vi "Main.vi"(8 "error in":errorcluster, 11 "Test Timer in":refnum<class "Test Timer.lvclass">) -> (0 "error out":errorcluster, 3 "Test Timer out":refnum<class "Test Timer.lvclass">)   [LabVIEW 2021, in "Test Timer.lvclass"]
doc: "The <b>Queued Message Handler</b> of the Worker that owns this VI."
uses:
  Test Timer.lvclass
  Test Timer.lvclass/Test Timer.ctl
  Initialization Data.ctl
  Response Cases.ctl
  Utility/Utility.lvlib
  Timer/Timer.lvclass
  <vilib>/addons/_Workers/Library/Case Label.ctl
  <vilib>/addons/_Workers/Library/Workers.lvlib
  Timer/rqp_Start.ctl
panel:
  in  "Exit":bool
  in  "Abort Timer":bool
  out "Response 2 recieved":i32
  out "Response 1 recieved":i32
  in  "Response case Test Timer":enum16{"Response 1", "Response 2"}(ring)
  in  "# Copies (0 = infinite repeat)":i32=3
  in  "Period [ms]":i32=1000 min=20
  in  "Start":bool
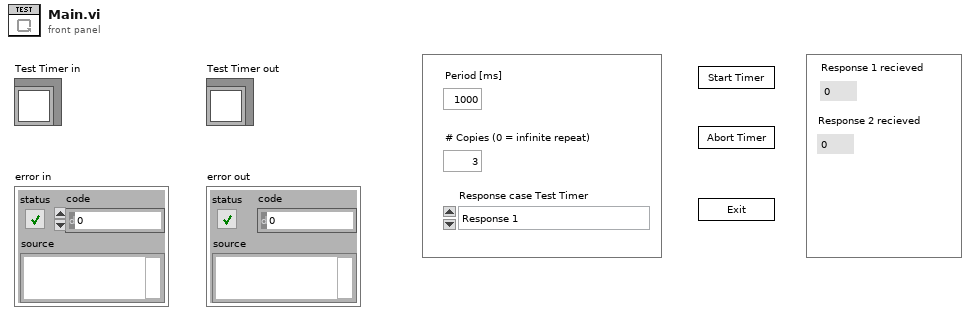
[diagram p1: front panel]
types:
  T1 = enum32{"Invalid", "Standard", "Closed", "Hidden", "Minimized", "Maximized"}
  T2 = typedef "Test Timer.lvclass/Initialization Data.ctl" = cluster{"Response Cases":T3}
  T3 = typedef "Test Timer.lvclass/Response Cases.ctl" = cluster{"Placeholder - Can be deleted":string}
  T4 = typedef "Timer.lvclass/rqp_Start.ctl" = cluster{"Timeout (ms)":i32, "# Copies":i32, "Response Case":T5}
  T5 = typedef "Workers.lvlib/Case Label.ctl" = string
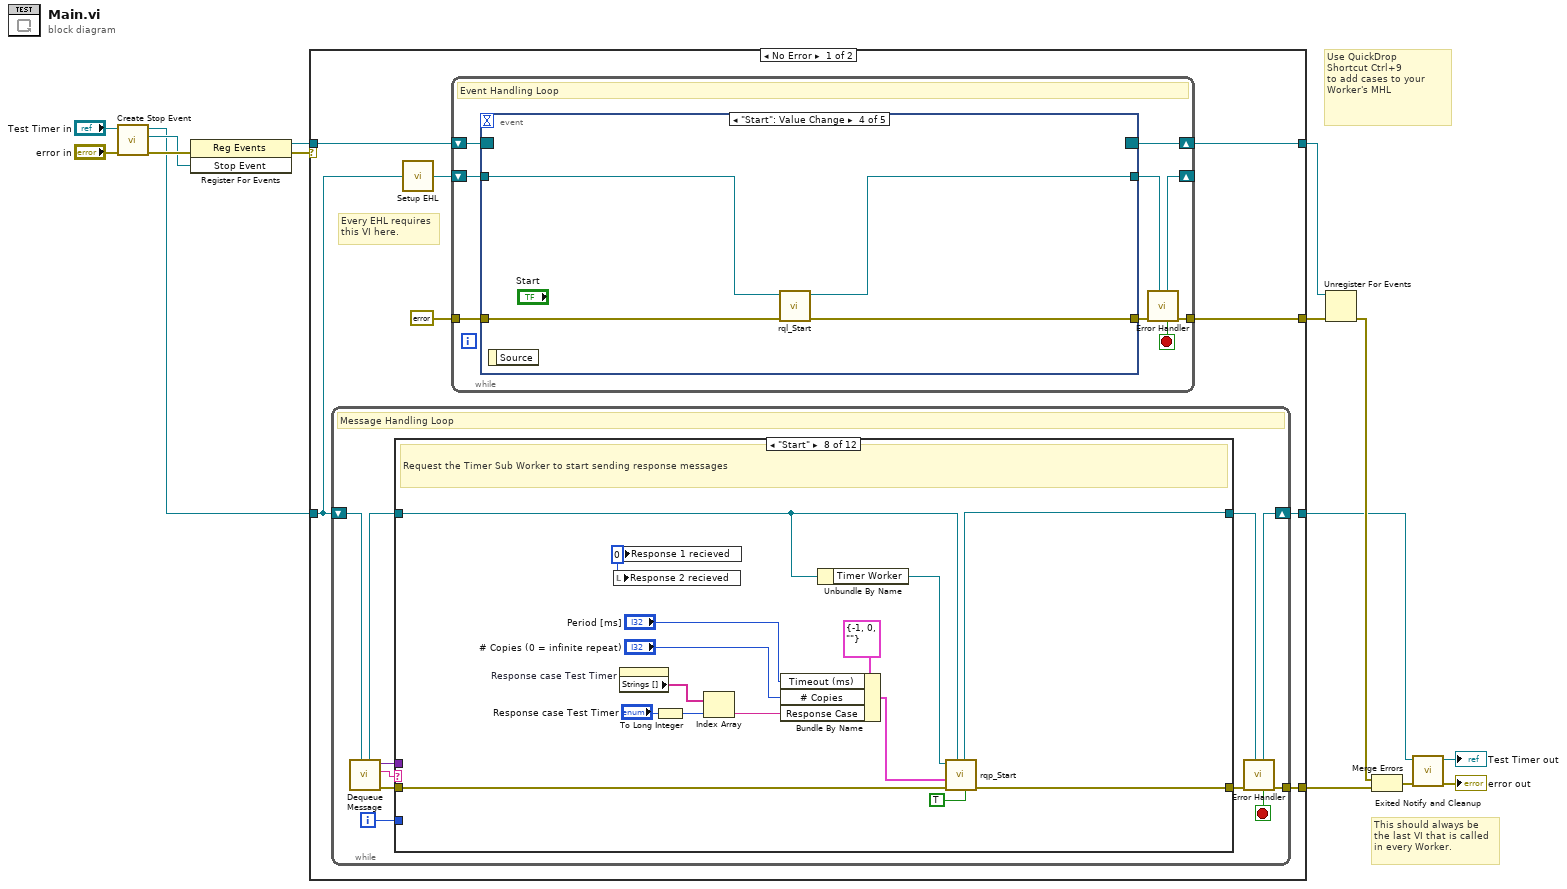
[diagram p0: block diagram]
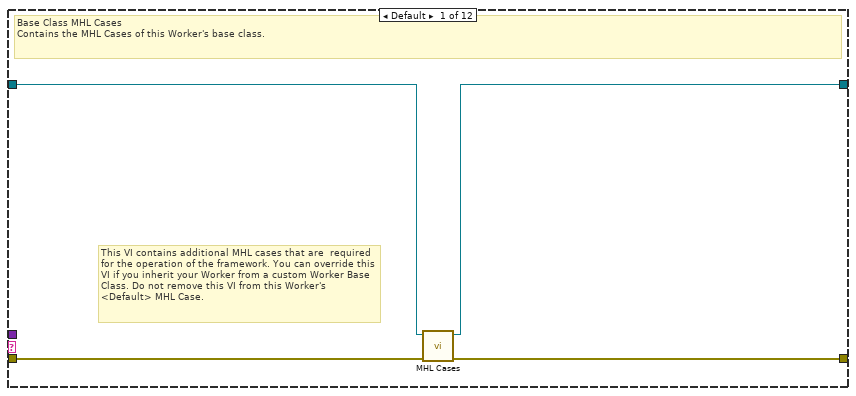
[diagram p2: hidden frame]
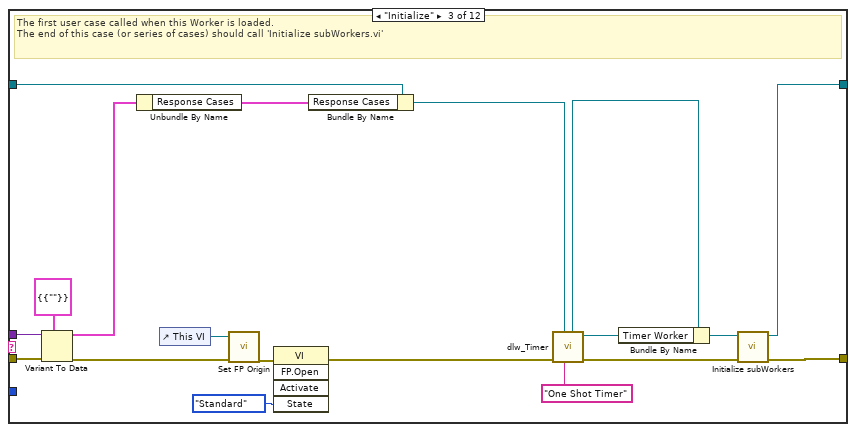
[diagram p4: hidden frame]
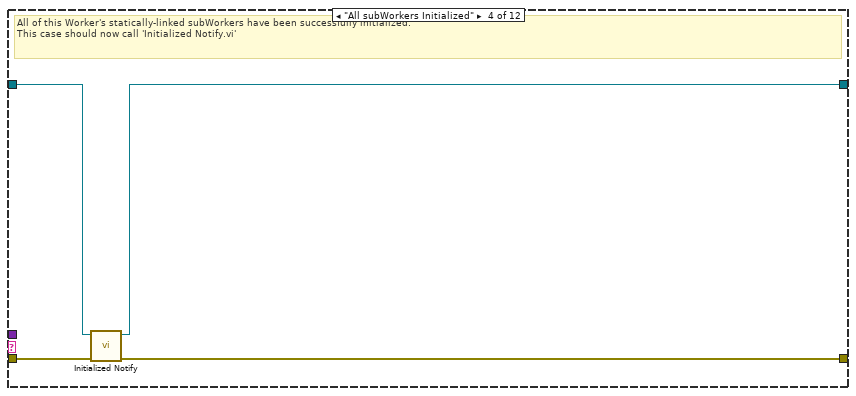
[diagram p5: hidden frame]
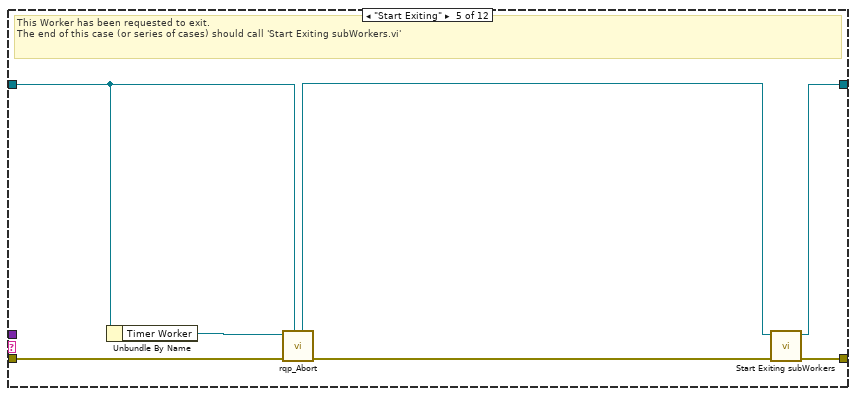
[diagram p6: hidden frame]
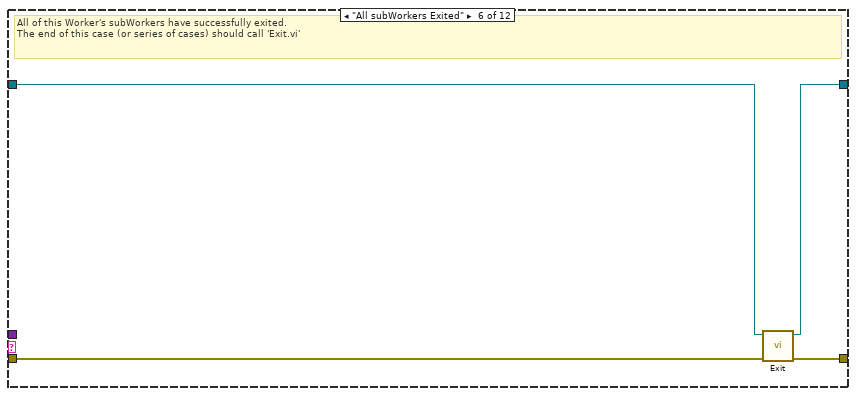
[diagram p7: hidden frame]
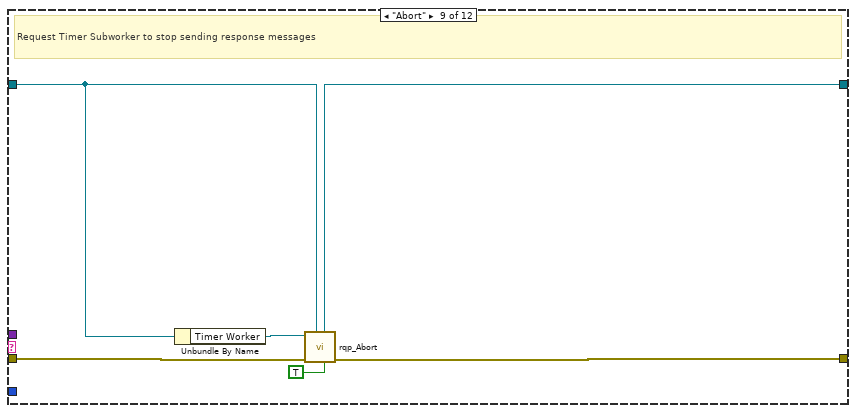
[diagram p9: hidden frame]
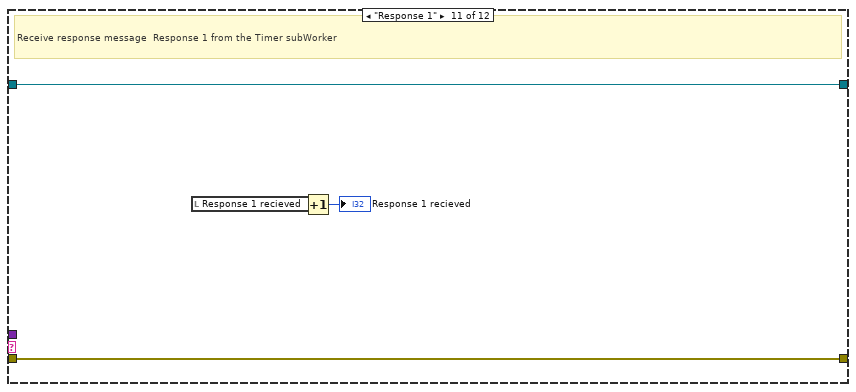
[diagram p11: hidden frame]
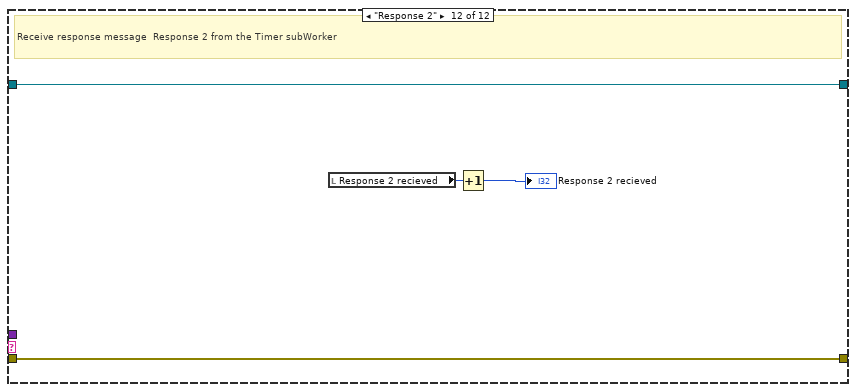
[diagram p12: hidden frame]
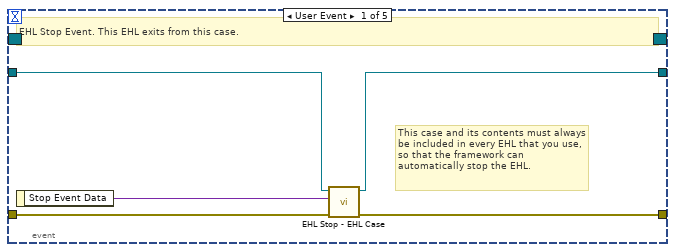
[diagram p13: hidden frame]
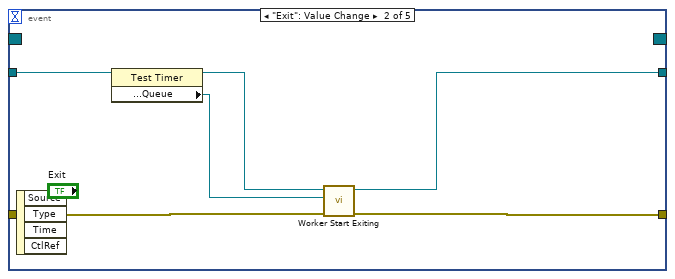
[diagram p14: hidden frame]
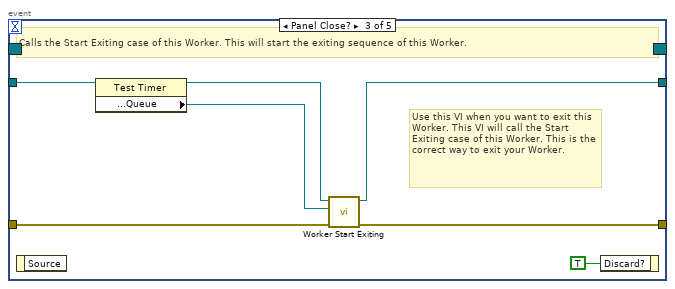
[diagram p15: hidden frame]
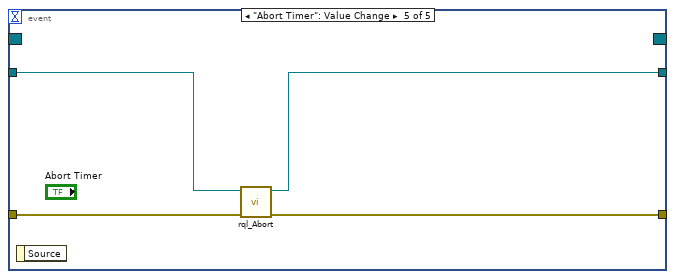
[diagram p16: hidden frame]
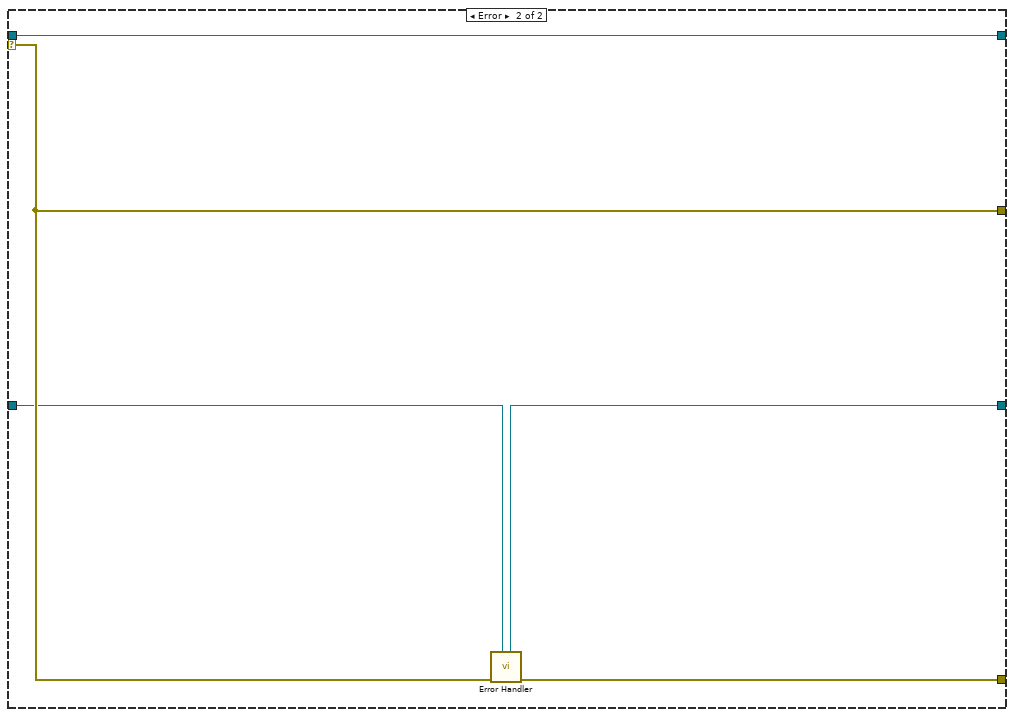
[diagram p17: hidden frame]
diagram:
  # "Use QuickDrop\nShortcut Ctrl+9\nto add cases to your\nWorker's MHL"
  # "This should always be the last VI that is called in every Worker."
  n1 = call-dynamic "Create Stop Event.vi"("error in"="error in", "Worker"="Test Timer in") -> ("error out"=w12:errorcluster, "Stop Event"=w4:refnum<user-event>, "Worker out"=w2:refnum<class "Test Timer.lvclass">)  [unwired: 7 in]
  n2 = register-events(error in=w12, w4) -> (reference out=w5:refnum<event-registration>, error out=w8:errorcluster)  [unwired: 1 in]
  n3 = case shown="No Error" w8 {
    tunnel: w2 -> [w17 w144]
    tunnel: [w21 w146] -> w11
    tunnel: w5 -> [w20 w145]
    tunnel: [w22 w147] -> w14
    tunnel: [w19 w145] -> w7
    tunnel: [w16 w143] -> w6
    selector: w8 -> [_ w147]
    frame No Error {
      # "Every EHL requires\nthis VI here."
      n4 = while {
        shift-right: [w30] -> w16
        shift-left: w17 -> [w31]
        tunnel: [w34] -> w21
        i -> [w25]
        stop <- w26 stop-if-true
        # "Message Handling Loop"
        n5 = call-dynamic "Dequeue Message.vi"("Worker"=w31) -> ("error out"=w33:errorcluster, "Case out"=w27:string, "Data out"=w24:variant, "Worker out"=w29:refnum<class "Test Timer.lvclass">)  [unwired: 6 in, 1 out]
        n6 = case "Worker MHL Case Structure (DO NOT CHANGE LABEL NAME)" shown="\"Start\"" w27 {
          tunnel: w33 -> [w38 w40 w58 w63 w67 w74 w76 w91 w96 w99 w103 w107]
          tunnel: [w37 w40 w59 w60 w70 w73 w76 w90 w97 w99 w103 w107] -> w32
          tunnel: w29 -> [w36 w39 w54 w62 w65 w72 w75 w78 w93 w98 w102 w106]
          tunnel: [w35 w39 w55 w61 w69 w71 w75 w79 w94 w98 w102 w106] -> w28
          tunnel: w25 -> [_ _ _ _ _ _ _ _ _ _ _ _]
          tunnel: w24 -> [_ _ w53 _ _ _ _ _ _ _ _ _]
          frame Default {
            # "This VI contains additional MHL cases that are  required for the operation of the framework. You can override this VI if you inherit your Worker from a custom Worker Base Class. Do not remove this VI from this Worker's <Default> MHL Case."
            # "Base Class MHL Cases\nContains the MHL Cases of this Worker's base class."
            n7 = call-dynamic "MHL Cases.vi"("error in"=w38, "Worker in"=w36) -> ("error out"=w37:errorcluster, "Worker out"=w35:refnum<class "Test Timer.lvclass">)  [unwired: 8 in]
          }
          frame "------------ FRAMEWORK CASES -----------" {
            # "Start of Workers Framework Cases"
          }
          frame "Initialize" {
            # "The first user case called when this Worker is loaded.\nThe end of this case (or series of cases) should call 'Initialize subWorkers.vi'"
            n8 = Variant To Data(error in=w58, type=T2 {"Response Cases"={"Placeholder - Can be deleted"=""}} ("Initialization Data"), Variant=w53) -> (data=w52:T2, error out=w57:errorcluster)
            n9 = Unbundle By Name(w52) -> ("Response Cases"=w51:T3)
            n10 = control-ref of="This VI"() -> (w49:refnum<vi>)
            n11 = call "Set FP Origin.vi"("error in"=w57, "VI ref in"=w49) -> ("error out"=w43:errorcluster)  [unwired: 8 in, 1 out]
            n12 = invoke class="VI" method="FP.Open"(error in=w43, "State"=T1."Standard") -> (error out=w41:errorcluster)  [unwired: 3 in, 4 out]
            n13 = Bundle By Name(cluster=w54, "Response Cases"=w51) -> (w48:refnum<class "Test Timer.lvclass">)
            n14 = call "dlw_Timer.vi"("Worker Alias"="One Shot Timer", "Caller in"=w48, "error in"=w41) -> ("error out"=w56:errorcluster, "Timer Out"=w45:refnum<class "Timer.lvclass">, "dup Caller out"=w47:refnum<class "Test Timer.lvclass">)  [unwired: 6 in]
            n15 = Bundle By Name(cluster=w47, "Timer Worker"=w45) -> (w46:refnum<class "Test Timer.lvclass">)
            n16 = call-dynamic "Initialize subWorkers.vi"("error in"=w56, "Worker"=w46) -> ("error out"=w59:errorcluster, "dup Worker out"=w55:refnum<class "Test Timer.lvclass">)  [unwired: 8 in]
          }
          frame "All subWorkers Initialized" {
            # "All of this Worker's statically-linked subWorkers have been successfully initialized.\nThis case should now call 'Initialized Notify.vi'"
            n17 = call-dynamic "Initialized Notify.vi"("error in"=w63, "Worker"=w62) -> ("error out"=w60:errorcluster, "dup Worker out"=w61:refnum<class "Test Timer.lvclass">)  [unwired: 8 in]
          }
          frame "Start Exiting" {
            # "This Worker has been requested to exit. \nThe end of this case (or series of cases) should call 'Start Exiting subWorkers.vi'"
            n18 = Unbundle By Name(w65) -> ("Timer Worker"=w64:refnum<class "Timer.lvclass">)
            n19 = call "rqp_Abort.vi"("Caller in"=w65, "error in"=w67, "Timer In"=w64) -> ("error out"=w68:errorcluster, "dup Caller out"=w66:refnum<class "Test Timer.lvclass">)  [unwired: 6 in, 1 out]
            n20 = call-dynamic "Start Exiting subWorkers.vi"("error_in"=w68, "Worker"=w66) -> ("error out"=w70:errorcluster, "dup Worker out"=w69:refnum<class "Test Timer.lvclass">)  [unwired: 8 in]
          }
          frame "All subWorkers Exited" {
            # "All of this Worker's subWorkers have successfully exited. \nThe end of this case (or series of cases) should call 'Exit.vi'"
            n21 = call-dynamic "Exit.vi"("error_in"=w74, "Worker"=w72) -> ("error out"=w73:errorcluster, "dup Worker out"=w71:refnum<class "Test Timer.lvclass">)  [unwired: 8 in]
          }
          frame "------------- LOCAL API CASES -------------" {
            # "Start of Workers Local API Cases"
          }
          frame "Start" {
            w80 = 0 ("# Response 1")
            # "Request the Timer Sub Worker to start sending response messages"
            n22 = local write "Response 2 recieved"(w80) -> ()
            n23 = local write "Response 1 recieved"(w80) -> ()
            n24 = property on="Response case Test Timer" class="Enum (strict)"() -> ("Strings []"=w84:string[])  [unwired: 2 in, 2 out]
            n25 = To Long Integer(number="Response case Test Timer") -> (32bit integer=w81:i32)
            n26 = Index Array(array=w84, index=w81) -> (element=w82:string)
            n27 = Bundle By Name(cluster=T4 {"Timeout (ms)"=-1, "# Copies"=0, "Response Case"=""} ("Data in"), "Timeout (ms)"="Period [ms]", "# Copies"="# Copies (0 = infinite repeat)", "Response Case"=w82) -> (w87:T4)
            n28 = Unbundle By Name(w78) -> ("Timer Worker"=w89:refnum<class "Timer.lvclass">)
            n29 = call "rqp_Start.vi"("Show in Debugger?"=TRUE, "Caller in"=w78, "error in"=w91, "Data in"=w87, "Timer In"=w89) -> ("error out"=w90:errorcluster, "dup Caller out"=w79:refnum<class "Test Timer.lvclass">)  [unwired: 4 in, 1 out]
          }
          frame "Abort" {
            # "Request Timer Subworker to stop sending response messages"
            n30 = Unbundle By Name(w93) -> ("Timer Worker"=w95:refnum<class "Timer.lvclass">)
            n31 = call "rqp_Abort.vi"("Show in Debugger?"=TRUE, "Caller in"=w93, "error in"=w96, "Timer In"=w95) -> ("error out"=w97:errorcluster, "dup Caller out"=w94:refnum<class "Test Timer.lvclass">)  [unwired: 5 in, 1 out]
          }
          frame "------------- RESPONSE CASES --------------" {
            # "Start of Workers Response Cases"
          }
          frame "Response 1" {
            # "Receive response message  Response 1 from the Timer subWorker"
            n32 = local read "Response 1 recieved"() -> (w100:i32)
            n33 = Increment(x=w100) -> (x+1=→"Response 1 recieved":i32)
          }
          frame "Response 2" {
            # "Receive response message  Response 2 from the Timer subWorker"
            n34 = local read "Response 2 recieved"() -> (w105:i32)
            n35 = Increment(x=w105) -> (x+1=→"Response 2 recieved":i32)
          }
        }
        n36 = call-dynamic "Error Handler.vi"("Worker"=w28, "error_in"=w32) -> ("error out"=w34:errorcluster, "Stop Loop"=w26:bool, "Worker out"=w30:refnum<class "Test Timer.lvclass">)  [unwired: 7 in]
      }
      n37 = call-dynamic "Setup EHL.vi"("Worker"=w17) -> ("Worker out"=w18:refnum<class "Test Timer.lvclass">)  [unwired: 14 in]
      n38 = while "Event Handling Loop" {
        shift-right: [w113] -> w19
        shift-left: w20 -> [w112]
        tunnel: [w114] -> w22
        tunnel: errorcluster {"status"=FALSE, "code"=0, "source"=""} ("error constant") -> [w116]
        shift-right: [w109] -> _
        shift-left: w18 -> [w111]
        stop <- w108 stop-if-true
        # "Event Handling Loop"
        n39 = event shown="[3] \"Start\": Value Change" {
          selector: w112 -> [_ _ _ _ _]
          dyn-events: [_ _ _ _ _] -> w113
          timeout: _ -> [_ _ _ _ _]
          tunnel: [w120 w127 w134 w138 w142] -> w115
          tunnel: w116 -> [w121 w126 w133 w137 w141]
          tunnel: w111 -> [w119 w123 w131 w135 w139]
          tunnel: [w118 w125 w130 w136 w140] -> w110
          event User Event {
            # "This case and its contents must always be included in every EHL that you use, so that the framework can automatically stop the EHL."
            # "EHL Stop Event. This EHL exits from this case."
            n40 = event-data() -> ("Stop Event Data"=w117:variant)  [unwired: 1 in]
            n41 = call-dynamic "EHL Stop - EHL Case.vi"("error in"=w121, "Stop Event Data"=w117, "Worker"=w119) -> ("error out"=w120:errorcluster, "Worker out"=w118:refnum<class "Test Timer.lvclass">)  [unwired: 7 in]
          }
          event "Exit": Value Change {
            n42 = event-data() -> ()  [unwired: 1 in, 4 out]
            n43 = property class="Test Timer"(reference=w123) -> (reference out=w124:refnum<class "Test Timer.lvclass">, "Accessors:Read:Public API:Queue"=w122:refnum<class "Message Queue.lvclass">)  [unwired: 1 in, 1 out]
            n44 = call-dynamic "Worker Start Exiting.vi"("error_in"=w126, "Message Queue"=w122, "Worker"=w124) -> ("error out"=w127:errorcluster, "dup Worker out"=w125:refnum<class "Test Timer.lvclass">)  [unwired: 7 in]
          }
          event Panel Close? {
            # "Use this VI when you want to exit this Worker. This VI will call the Start Exiting case of this Worker. This is the correct way to exit your Worker."
            # "Calls the Start Exiting case of this Worker. This will start the exiting sequence of this Worker."
            n45 = event-data() -> ()  [unwired: 1 in, 1 out]
            n46 = property class="Test Timer"(reference=w131) -> (reference out=w129:refnum<class "Test Timer.lvclass">, "Accessors:Read:Public API:Queue"=w128:refnum<class "Message Queue.lvclass">)  [unwired: 1 in, 1 out]
            n47 = call-dynamic "Worker Start Exiting.vi"("error_in"=w133, "Message Queue"=w128, "Worker"=w129) -> ("error out"=w134:errorcluster, "dup Worker out"=w130:refnum<class "Test Timer.lvclass">)  [unwired: 7 in]
            n48 = event-data("Discard?"=TRUE) -> ()  [unwired: 1 in, 1 out]
          }
          event "Start": Value Change {
            n49 = event-data() -> ()  [unwired: 1 in, 1 out]
            n50 = call "rql_Start.vi"("error in"=w137, "Test Timer in"=w135) -> ("error out"=w138:errorcluster, "dup Test Timer out"=w136:refnum<class "Test Timer.lvclass">)  [unwired: 8 in]
          }
          event "Abort Timer": Value Change {
            n51 = event-data() -> ()  [unwired: 1 in, 1 out]
            n52 = call "rql_Abort.vi"("error in"=w141, "Test Timer in"=w139) -> ("error out"=w142:errorcluster, "dup Test Timer out"=w140:refnum<class "Test Timer.lvclass">)  [unwired: 8 in]
          }
        }
        n53 = call-dynamic "Error Handler.vi"("Worker"=w110, "error_in"=w115) -> ("error out"=w114:errorcluster, "Stop Loop"=w108:bool, "Worker out"=w109:refnum<class "Test Timer.lvclass">)  [unwired: 7 in]
      }
    }
    frame Error {
      n54 = call-dynamic "Error Handler.vi"("Worker"=w144, "error_in"=w147) -> ("error out"=w146:errorcluster, "Worker out"=w143:refnum<class "Test Timer.lvclass">)  [unwired: 7 in, 1 out]
    }
  }
  n55 = Unregister For Events(event registration refnum=w7, error in=w14) -> (error out=w15:errorcluster)
  n56 = Merge Errors(w15, w11) -> (w13:errorcluster)
  n57 = call-dynamic "Exited Notify and Cleanup.vi"("error_in"=w13, "Worker"=w6) -> ("error out"=→"error out":errorcluster, "dup Worker out"=→"Test Timer out":refnum<class "Test Timer.lvclass">)  [unwired: 8 in]
